vi "Coerce Value.vi"(8 "error in (no error)":errorcluster, 9 "Value":variant, 10 "ParamTags":T1, 11 "Rigol DG822 Square in":refnum<class "Rigol DG822 Square.lvclass">) -> (0 "error out":errorcluster, 1 "Coerced Value":variant, 3 "Rigol DG822 Square out":refnum<class "Rigol DG822 Square.lvclass">)   [LabVIEW 2021, in "Rigol DG822 UI.lvlib" / "Rigol DG822 Square.lvlib" / "Rigol DG822 Square.lvclass"]
uses:
  Rigol DG822 Square.lvclass
  Rigol DG822 UI/lib/controls.llb/WaveformParamTags.ctl
  Rigol DG822 UI/lib/controls.llb/FreqUnit.ctl
  Rigol DG822 UI/lib/controls.llb/PeriodUnit.ctl
  Rigol DG822 Square.lvclass/Rigol DG822 Square.ctl
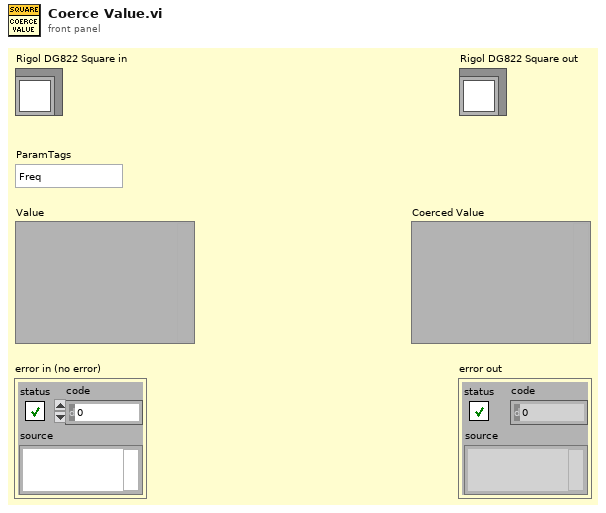
[diagram p1: front panel]
types:
  T1 = typedef "WaveformParamTags.ctl" = enum16{"Freq", "Period", "Ampl", "HighL", "Offset", "LowL", "Phase", "Duty", "Width", "RisEdge", "FallEdge"}
  T2 = typedef "FreqUnit.ctl" = enum32{"No Selection", "MHz", "kHz", "Hz", "mHz", "uHz"}
  T3 = cluster{"Freq":dbl, "FreqUnit":T2, "FreqUnitPrecision":dbl}
  T4 = typedef "PeriodUnit.ctl" = enum32{"No Selection", "s", "ms", "us", "ns"}
  T5 = cluster{"Period":dbl, "PeriodUnit":T4, "PeriodUnitPrecision":dbl}
  T6 = cluster{"Ampl":dbl, "AmplUnit":enum32{"No Selection", "Vpp", "mVpp"}, "AmplUnitPrecision":dbl}
  T7 = cluster{"HighL":dbl, "HighLUnit":enum32{"No Selection", "V", "mV"}, "HighLUnitPrecision":dbl}
  T8 = cluster{"Offset":dbl, "OffsetUnit":enum32{"No Selection", "Vdc", "mVdc"}, "OffsetUnitPrecision":dbl}
  T9 = cluster{"LowL":dbl, "LowLUnit":enum32{"No Selection", "V", "mV"}, "LowLUnitPrecision":dbl}
  T10 = cluster{"Phase":dbl, "PhaseUnit":enum32{"°"}, "PhaseUnitPrecision":dbl}
  T11 = cluster{"Duty":dbl, "DutyUnit":enum32{"%"}, "DutyUnitPrcs":dbl}
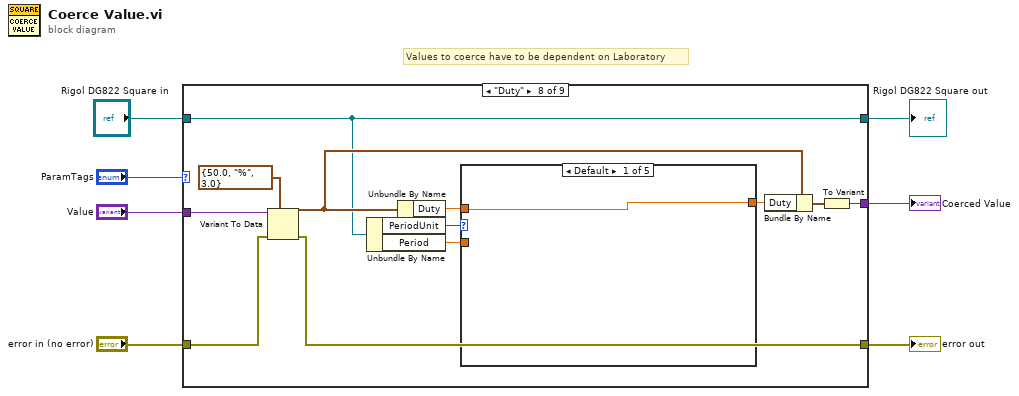
[diagram p0: block diagram]
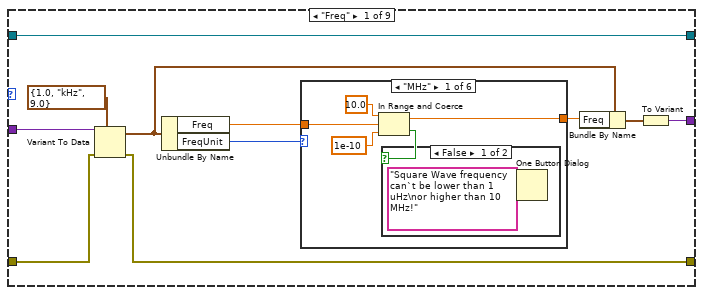
[diagram p2: hidden frame]
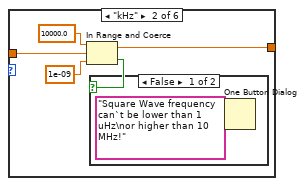
[diagram p4: hidden frame]
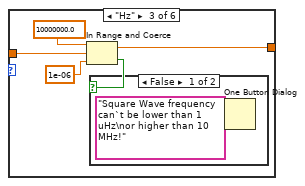
[diagram p6: hidden frame]
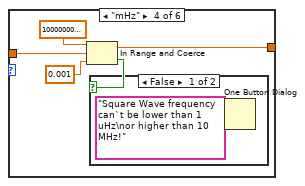
[diagram p8: hidden frame]
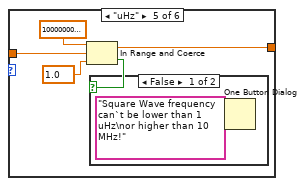
[diagram p10: hidden frame]
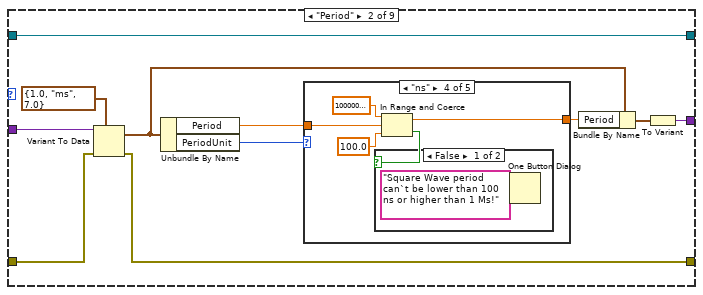
[diagram p13: hidden frame]
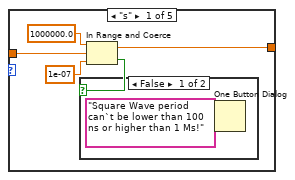
[diagram p14: hidden frame]
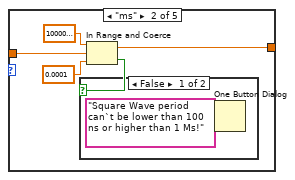
[diagram p16: hidden frame]
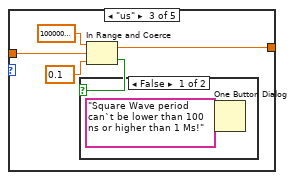
[diagram p18: hidden frame]
diagram:
  # "Values to coerce have to be dependent on Laboratory"
  n1 = case shown="\"Duty\"" "ParamTags" {
    tunnel: "Value" -> [w14 w57 w93 w119 w167 w233 w279 w296 w362]
    tunnel: "error in (no error)" -> [w12 w53 w90 w117 w165 w231 w276 w294 w361]
    tunnel: [w11 w52 w89 w116 w164 w230 w275 w293 w361] -> w4
    tunnel: [w9 w50 w87 w114 w162 w228 w273 w291 w362] -> w1
    tunnel: "Rigol DG822 Square in" -> [w8 w54 w91 w112 w160 w227 w277 w289 w363]
    tunnel: [w8 w54 w91 w112 w160 w227 w277 w289 w363] -> w2
    frame "Freq" {
      n2 = Variant To Data(error in=w12, type=T3 {"Freq"=1.0, "FreqUnit"=enum."kHz", "FreqUnitPrecision"=9.0} ("Freq"), Variant=w14) -> (data=w13:T3, error out=w11:errorcluster)
      n3 = Unbundle By Name(w13) -> ("Freq"=w17:dbl, "FreqUnit"=w18:T2)
      n4 = case shown="\"MHz\"" w18 {
        tunnel: [w20 w26 w32 w38 w44 w49] -> w16
        tunnel: w17 -> [w21 w27 w33 w39 w45 w49]
        frame "MHz" {
          n5 = In Range and Coerce(upper limit=10.0, x=w21, lower limit=1e-10 ("t")) -> (coerced(x)=w20:dbl, In Range?=w19:bool)
          n6 = case shown="False" w19 {
            frame False {
              n7 = One Button Dialog(message="Square Wave frequency can`t be lower than 1 uHz\nor higher than 10 MHz!") -> ()  [unwired: 1 in, 1 out]
            }
            frame True {
            }
          }
        }
        frame "kHz" {
          n8 = In Range and Coerce(upper limit=10000.0, x=w27, lower limit=1e-09 ("t")) -> (coerced(x)=w26:dbl, In Range?=w25:bool)
          n9 = case shown="False" w25 {
            frame False {
              n10 = One Button Dialog(message="Square Wave frequency can`t be lower than 1 uHz\nor higher than 10 MHz!") -> ()  [unwired: 1 in, 1 out]
            }
            frame True {
            }
          }
        }
        frame "Hz" {
          n11 = In Range and Coerce(upper limit=10000000.0, x=w33, lower limit=1e-06 ("t")) -> (coerced(x)=w32:dbl, In Range?=w31:bool)
          n12 = case shown="False" w31 {
            frame False {
              n13 = One Button Dialog(message="Square Wave frequency can`t be lower than 1 uHz\nor higher than 10 MHz!") -> ()  [unwired: 1 in, 1 out]
            }
            frame True {
            }
          }
        }
        frame "mHz" {
          n14 = In Range and Coerce(upper limit=10000000000.0, x=w39, lower limit=0.001 ("t")) -> (coerced(x)=w38:dbl, In Range?=w37:bool)
          n15 = case shown="False" w37 {
            frame False {
              n16 = One Button Dialog(message="Square Wave frequency can`t be lower than 1 uHz\nor higher than 10 MHz!") -> ()  [unwired: 1 in, 1 out]
            }
            frame True {
            }
          }
        }
        frame "uHz" {
          n17 = In Range and Coerce(upper limit=10000000000000.0, x=w45, lower limit=1.0 ("t")) -> (coerced(x)=w44:dbl, In Range?=w43:bool)
          n18 = case shown="False" w43 {
            frame False {
              n19 = One Button Dialog(message="Square Wave frequency can`t be lower than 1 uHz\nor higher than 10 MHz!") -> ()  [unwired: 1 in, 1 out]
            }
            frame True {
            }
          }
        }
        frame Default {
        }
      }
      n20 = Bundle By Name(cluster=w13, "Freq"=w16) -> (w10:T3)
      n21 = To Variant(anything=w10) -> (Variant=w9:variant)
    }
    frame "Period" {
      n22 = Variant To Data(error in=w53, type=T5 {"Period"=1.0, "PeriodUnit"=enum."ms", "PeriodUnitPrecision"=7.0} ("Period"), Variant=w57) -> (data=w56:T5, error out=w52:errorcluster)
      n23 = Unbundle By Name(w56) -> ("Period"=w59:dbl, "PeriodUnit"=w60:T4)
      n24 = case shown="\"ns\"" w60 {
        tunnel: [w62 w68 w74 w80 w85] -> w58
        tunnel: w59 -> [w63 w69 w75 w81 w85]
        frame "s" {
          n25 = In Range and Coerce(upper limit=1000000.0, x=w63, lower limit=1e-07 ("t")) -> (coerced(x)=w62:dbl, In Range?=w61:bool)
          n26 = case shown="False" w61 {
            frame False {
              n27 = One Button Dialog(message="Square Wave period can`t be lower than 100 ns or higher than 1 Ms!") -> ()  [unwired: 1 in, 1 out]
            }
            frame True {
            }
          }
        }
        frame "ms" {
          n28 = In Range and Coerce(upper limit=1000000000.0, x=w69, lower limit=0.0001 ("t")) -> (coerced(x)=w68:dbl, In Range?=w67:bool)
          n29 = case shown="False" w67 {
            frame False {
              n30 = One Button Dialog(message="Square Wave period can`t be lower than 100 ns or higher than 1 Ms!") -> ()  [unwired: 1 in, 1 out]
            }
            frame True {
            }
          }
        }
        frame "us" {
          n31 = In Range and Coerce(upper limit=1000000000000.0, x=w75, lower limit=0.1 ("t")) -> (coerced(x)=w74:dbl, In Range?=w73:bool)
          n32 = case shown="False" w73 {
            frame False {
              n33 = One Button Dialog(message="Square Wave period can`t be lower than 100 ns or higher than 1 Ms!") -> ()  [unwired: 1 in, 1 out]
            }
            frame True {
            }
          }
        }
        frame "ns" {
          n34 = In Range and Coerce(upper limit=1000000000000000.0, x=w81, lower limit=100.0 ("t")) -> (coerced(x)=w80:dbl, In Range?=w79:bool)
          n35 = case shown="False" w79 {
            frame False {
              n36 = One Button Dialog(message="Square Wave period can`t be lower than 100 ns or higher than 1 Ms!") -> ()  [unwired: 1 in, 1 out]
            }
            frame True {
            }
          }
        }
        frame Default {
        }
      }
      n37 = Bundle By Name(cluster=w56, "Period"=w58) -> (w51:T5)
      n38 = To Variant(anything=w51) -> (Variant=w50:variant)
    }
    frame "Ampl" {
      n39 = Variant To Data(error in=w90, type=T6 {"Ampl"=5.0, "AmplUnit"=enum."Vpp", "AmplUnitPrecision"=4.0} ("Ampl"), Variant=w93) -> (data=w92:T6, error out=w89:errorcluster)
      n40 = Unbundle By Name(w92) -> ("Ampl"=w95:dbl, "AmplUnit"=w96:enum32{"No Selection", "Vpp", "mVpp"})
      n41 = case shown="\"Vpp\"" w96 {
        tunnel: [w99 w105 w109] -> w94
        tunnel: w95 -> [w100 w106 w109]
        frame "Vpp" {
          n42 = In Range and Coerce(upper limit=10.0, x=w100, lower limit=0.002 ("t")) -> (coerced(x)=w99:dbl, In Range?=w97:bool)
          n43 = case shown="False" w97 {
            frame False {
              n44 = One Button Dialog(message="Amplitude can`t be lower than 2 mVpp\nor higher than 10 Vpp!") -> ()  [unwired: 1 in, 1 out]
            }
            frame True {
            }
          }
        }
        frame "mVpp" {
          n45 = In Range and Coerce(upper limit=10000.0, x=w106, lower limit=2.0 ("t")) -> (coerced(x)=w105:dbl, In Range?=w103:bool)
          n46 = case shown="False" w103 {
            frame False {
              n47 = One Button Dialog(message="Amplitude can`t be lower than 2 mVpp\nor higher than 10 Vpp!") -> ()  [unwired: 1 in, 1 out]
            }
            frame True {
            }
          }
        }
        frame Default {
        }
      }
      n48 = Bundle By Name(cluster=w92, "Ampl"=w94) -> (w88:T6)
      n49 = To Variant(anything=w88) -> (Variant=w87:variant)
    }
    frame "HighL" {
      n50 = Variant To Data(error in=w117, type=T7 {"HighL"=2.5, "HighLUnit"=enum."V", "HighLUnitPrecision"=4.0} ("HighL"), Variant=w119) -> (data=w118:T7, error out=w116:errorcluster)
      n51 = Unbundle By Name(w118) -> ("HighL"=w121:dbl, "HighLUnit"=w122:enum32{"No Selection", "V", "mV"})
      n52 = Unbundle By Name(w112) -> ("LowL"=w111:dbl, "LowLUnit"=w110:enum32{"No Selection", "V", "mV"})
      n53 = case shown="\"V\"" w122 {
        tunnel: [w127 w144 w157] -> w120
        tunnel: w121 -> [w128 w145 w157]
        tunnel: w111 -> [w123 w140 _]
        tunnel: w110 -> [w125 w142 _]
        frame "V" {
          n54 = case shown="\"V\"" w125 {
            tunnel: [w130 w136 w138] -> w124
            tunnel: w123 -> [w132 w137 w138]
            frame "V" {
              n55 = Add(x=w132, y=0.002 ("upper limit")) -> (x+y=w130:dbl)
            }
            frame "mV" {
              n56 = Divide(x=w137, y=1000.0) -> (x/y=w135:dbl)
              n57 = Add(x=w135, y=0.002 ("upper limit")) -> (x+y=w136:dbl)
            }
            frame Default {
            }
          }
          n58 = In Range and Coerce(upper limit=5.0, x=w128, lower limit=w124) -> (coerced(x)=w127:dbl, In Range?=w126:bool)
          n59 = case shown="False" w126 {
            frame False {
              n60 = One Button Dialog(message="HighL can`t be higher than 5 V or less than 2 mV higher than LowL!\n") -> ()  [unwired: 1 in, 1 out]
            }
            frame True {
            }
          }
        }
        frame "mV" {
          n61 = case shown="\"mV\"" w142 {
            tunnel: [w150 w154 w155] -> w141
            tunnel: w140 -> [w149 w152 w155]
            frame "V" {
              n62 = Multiply(x=w149, y=1000.0) -> (x*y=w147:dbl)
              n63 = Add(x=w147, y=2.0 ("upper limit")) -> (x+y=w150:dbl)
            }
            frame "mV" {
              n64 = Add(x=w152, y=2.0 ("upper limit")) -> (x+y=w154:dbl)
            }
            frame Default {
            }
          }
          n65 = In Range and Coerce(upper limit=5000.0, x=w145, lower limit=w141) -> (coerced(x)=w144:dbl, In Range?=w143:bool)
          n66 = case shown="False" w143 {
            frame False {
              n67 = One Button Dialog(message="HighL can`t be higher than 5 V or less than 2 mV higher than LowL!\n") -> ()  [unwired: 1 in, 1 out]
            }
            frame True {
            }
          }
        }
        frame Default {
        }
      }
      n68 = Bundle By Name(cluster=w118, "HighL"=w120) -> (w115:T7)
      n69 = To Variant(anything=w115) -> (Variant=w114:variant)
    }
    frame "Offset" {
      n70 = Variant To Data(error in=w165, type=T8 {"Offset"=0.0, "OffsetUnit"=enum."Vdc", "OffsetUnitPrecision"=4.0} ("Offset"), Variant=w167) -> (data=w166:T8, error out=w164:errorcluster)
      n71 = Unbundle By Name(w166) -> ("Offset"=w169:dbl, "OffsetUnit"=w170:enum32{"No Selection", "Vdc", "mVdc"})
      n72 = Unbundle By Name(w160) -> ("Ampl"=w159:dbl, "AmplUnit"=w158:enum32{"No Selection", "Vpp", "mVpp"})
      n73 = case shown="\"mVdc\"" w170 {
        tunnel: [w176 w202 w223] -> w168
        tunnel: w169 -> [w177 w203 w223]
        tunnel: w159 -> [w173 w199 _]
        tunnel: w158 -> [w174 w200 _]
        frame "Vdc" {
          n74 = case shown="\"Vpp\"" w174 {
            tunnel: w173 -> [w184 w192 _]
            tunnel: [w179 w187 5.0] -> w172
            tunnel: [w178 w186 -5.0] -> w171
            frame "Vpp" {
              w180 = 2.0 ("t")
              n75 = Add(x=w184, y=-10.0 ("t")) -> (x+y=w182:dbl)
              n76 = Subtract(x=10.0 ("t"), y=w184) -> (x-y=w181:dbl)
              n77 = Divide(x=w182, y=w180) -> (x/y=w178:dbl)
              n78 = Divide(x=w181, y=w180) -> (x/y=w179:dbl)
            }
            frame "mVpp" {
              w188 = 2000.0 ("t")
              n79 = Add(x=w192, y=-10000.0 ("t")) -> (x+y=w190:dbl)
              n80 = Subtract(x=10000.0 ("t"), y=w192) -> (x-y=w189:dbl)
              n81 = Divide(x=w190, y=w188) -> (x/y=w186:dbl)
              n82 = Divide(x=w189, y=w188) -> (x/y=w187:dbl)
            }
            frame Default {
            }
          }
          n83 = In Range and Coerce(upper limit=w172, x=w177, lower limit=w171) -> (coerced(x)=w176:dbl, In Range?=w175:bool)
          n84 = case shown="False" w175 {
            frame False {
              n85 = One Button Dialog(message="Offset upper and lower limit can`t exceed (10 - Ampl)/2 value") -> ()  [unwired: 1 in, 1 out]
            }
            frame True {
            }
          }
        }
        frame "mVdc" {
          n86 = case shown="\"Vpp\"" w200 {
            tunnel: w199 -> [w210 w218 _]
            tunnel: [w205 w213 5.0] -> w198
            tunnel: [w204 w212 -5.0] -> w197
            frame "Vpp" {
              w206 = 0.002 ("t")
              n87 = Add(x=w210, y=-10.0 ("t")) -> (x+y=w208:dbl)
              n88 = Subtract(x=10.0 ("t"), y=w210) -> (x-y=w207:dbl)
              n89 = Divide(x=w208, y=w206) -> (x/y=w204:dbl)
              n90 = Divide(x=w207, y=w206) -> (x/y=w205:dbl)
            }
            frame "mVpp" {
              w214 = 2.0 ("t")
              n91 = Add(x=w218, y=-10000.0 ("t")) -> (x+y=w216:dbl)
              n92 = Subtract(x=10000.0 ("t"), y=w218) -> (x-y=w215:dbl)
              n93 = Divide(x=w216, y=w214) -> (x/y=w212:dbl)
              n94 = Divide(x=w215, y=w214) -> (x/y=w213:dbl)
            }
            frame Default {
            }
          }
          n95 = In Range and Coerce(upper limit=w198, x=w203, lower limit=w197) -> (coerced(x)=w202:dbl, In Range?=w201:bool)
          n96 = case shown="False" w201 {
            frame False {
              n97 = One Button Dialog(message="Offset upper and lower limit can`t exceed (10 - Ampl)/2 value") -> ()  [unwired: 1 in, 1 out]
            }
            frame True {
            }
          }
        }
        frame Default {
        }
      }
      n98 = Bundle By Name(cluster=w166, "Offset"=w168) -> (w163:T8)
      n99 = To Variant(anything=w163) -> (Variant=w162:variant)
    }
    frame "LowL" {
      n100 = Variant To Data(error in=w231, type=T9 {"LowL"=-2.5, "LowLUnit"=enum."V", "LowLUnitPrecision"=4.0} ("LowL"), Variant=w233) -> (data=w232:T9, error out=w230:errorcluster)
      n101 = Unbundle By Name(w232) -> ("LowL"=w235:dbl, "LowLUnit"=w236:enum32{"No Selection", "V", "mV"})
      n102 = Unbundle By Name(w227) -> ("HighL"=w226:dbl, "HighLUnit"=w225:enum32{"No Selection", "V", "mV"})
      n103 = case shown="\"mV\"" w236 {
        tunnel: [w242 w259 w271] -> w234
        tunnel: w235 -> [w243 w260 w271]
        tunnel: w226 -> [w239 w256 _]
        tunnel: w225 -> [w240 w257 _]
        frame "V" {
          n104 = case shown="\"mV\"" w240 {
            tunnel: [w244 w250 w252] -> w237
            tunnel: w239 -> [w246 w251 w252]
            frame "V" {
              n105 = Subtract(x=w246, y=0.002 ("upper limit")) -> (x-y=w244:dbl)
            }
            frame "mV" {
              n106 = Divide(x=w251, y=1000.0) -> (x/y=w249:dbl)
              n107 = Subtract(x=w249, y=0.002 ("upper limit")) -> (x-y=w250:dbl)
            }
            frame Default {
            }
          }
          n108 = In Range and Coerce(upper limit=w237, x=w243, lower limit=-5.0 ("upper limit")) -> (coerced(x)=w242:dbl, In Range?=w241:bool)
          n109 = case shown="False" w241 {
            frame False {
              n110 = One Button Dialog(message="LowL can`t be lower  than -5 V or less than 2 mV lower than HighL!") -> ()  [unwired: 1 in, 1 out]
            }
            frame True {
            }
          }
        }
        frame "mV" {
          n111 = case shown="\"V\"" w257 {
            tunnel: [w264 w268 w269] -> w254
            tunnel: w256 -> [w263 w266 w269]
            frame "V" {
              n112 = Multiply(x=w263, y=1000.0) -> (x*y=w261:dbl)
              n113 = Subtract(x=w261, y=2.0 ("upper limit")) -> (x-y=w264:dbl)
            }
            frame "mV" {
              n114 = Subtract(x=w266, y=2.0 ("upper limit")) -> (x-y=w268:dbl)
            }
            frame Default {
            }
          }
          n115 = In Range and Coerce(upper limit=w254, x=w260, lower limit=-5000.0 ("upper limit")) -> (coerced(x)=w259:dbl, In Range?=w258:bool)
          n116 = case shown="False" w258 {
            frame False {
              n117 = One Button Dialog(message="LowL can`t be lower  than -5 V or less than 2 mV lower than HighL!") -> ()  [unwired: 1 in, 1 out]
            }
            frame True {
            }
          }
        }
        frame Default {
        }
      }
      n118 = Bundle By Name(cluster=w232, "LowL"=w234) -> (w229:T9)
      n119 = To Variant(anything=w229) -> (Variant=w228:variant)
    }
    frame "Phase" {
      n120 = Variant To Data(error in=w276, type=T10 {"Phase"=0.0, "PhaseUnit"=enum."°", "PhaseUnitPrecision"=3.0} ("Phase"), Variant=w279) -> (data=w278:T10, error out=w275:errorcluster)
      n121 = Unbundle By Name(w278) -> ("Phase"=w281:dbl, "PhaseUnit"=w282:enum32{"°"})
      n122 = case shown="\"°\"" w282 {
        tunnel: [w283 w284] -> w280
        tunnel: w281 -> [w283 w285]
        frame Default {
        }
        frame "°" {
          n123 = Quotient & Remainder(x=w285, y=360.0) -> (x-y*floor(x/y)=w284:dbl)  [unwired: 1 out]
        }
      }
      n124 = Bundle By Name(cluster=w278, "Phase"=w280) -> (w274:T10)
      n125 = To Variant(anything=w274) -> (Variant=w273:variant)
    }
    frame "Duty" {
      n126 = Variant To Data(error in=w294, type=T11 {"Duty"=50.0, "DutyUnit"=enum."%", "DutyUnitPrcs"=3.0} ("Duty"), Variant=w296) -> (data=w295:T11, error out=w293:errorcluster)
      n127 = Unbundle By Name(w289) -> ("PeriodUnit"=w288:enum32{"No Selection", "s", "ms", "us", "ns"}, "Period"=w287:dbl)
      n128 = Unbundle By Name(w295) -> ("Duty"=w298:dbl)
      n129 = case shown="Default" w288 {
        tunnel: [w299 w308 w325 w342 w354] -> w297
        tunnel: w298 -> [w299 w307 w324 w341 w353]
        tunnel: w287 -> [_ w302 w319 w336 _]
        frame Default {
        }
        frame "ns" {
          w301 = 2000.0 ("lower limit")
          n130 = Multiply(x=100.0 ("y"), y=w302) -> (x*y=w309:dbl)
          n131 = Multiply(x=w307, y=w302) -> (x*y=w311:dbl)
          n132 = Divide(x=w301, y=w302) -> (x/y=w303:dbl)
          n133 = Subtract(x=w309, y=w301) -> (x-y=w300:dbl)
          n134 = Divide(x=w300, y=w302) -> (x/y=w304:dbl)
          n135 = In Range and Coerce(upper limit=w300, x=w311, lower limit=w301) -> (coerced(x)=w310:dbl, In Range?=w305:bool)
          n136 = case shown="False" w305 {
            tunnel: w303 -> [w315 _]
            tunnel: w304 -> [w312 _]
            frame False {
              w313 = "%" ("input 2")
              n137 = Format Into String(format string="Duty Cycle can`t be lower than %.3f %s\nor higher than %.3f %s!" ("message"), w315, w313, w312, w313) -> (resulting string=w316:string)  [unwired: 2 in, 1 out]
              n138 = One Button Dialog(message=w316) -> ()  [unwired: 1 in, 1 out]
            }
            frame True {
            }
          }
          n139 = Divide(x=w310, y=w302) -> (x/y=w308:dbl)
        }
        frame "us" {
          w318 = 2.0 ("lower limit")
          n140 = Multiply(x=100.0 ("y"), y=w319) -> (x*y=w326:dbl)
          n141 = Multiply(x=w324, y=w319) -> (x*y=w328:dbl)
          n142 = Divide(x=w318, y=w319) -> (x/y=w320:dbl)
          n143 = Subtract(x=w326, y=w318) -> (x-y=w317:dbl)
          n144 = Divide(x=w317, y=w319) -> (x/y=w321:dbl)
          n145 = In Range and Coerce(upper limit=w317, x=w328, lower limit=w318) -> (coerced(x)=w327:dbl, In Range?=w322:bool)
          n146 = case shown="False" w322 {
            tunnel: w320 -> [w332 _]
            tunnel: w321 -> [w329 _]
            frame False {
              w330 = "%" ("input 2")
              n147 = Format Into String(format string="Duty Cycle can`t be lower than %.3f %s\nor higher than %.3f %s!" ("message"), w332, w330, w329, w330) -> (resulting string=w333:string)  [unwired: 2 in, 1 out]
              n148 = One Button Dialog(message=w333) -> ()  [unwired: 1 in, 1 out]
            }
            frame True {
            }
          }
          n149 = Divide(x=w327, y=w319) -> (x/y=w325:dbl)
        }
        frame "ms" {
          w335 = 0.002 ("lower limit")
          n150 = Multiply(x=100.0 ("y"), y=w336) -> (x*y=w343:dbl)
          n151 = Multiply(x=w341, y=w336) -> (x*y=w345:dbl)
          n152 = Divide(x=w335, y=w336) -> (x/y=w337:dbl)
          n153 = Subtract(x=w343, y=w335) -> (x-y=w334:dbl)
          n154 = Divide(x=w334, y=w336) -> (x/y=w338:dbl)
          n155 = In Range and Coerce(upper limit=w334, x=w345, lower limit=w335) -> (coerced(x)=w344:dbl, In Range?=w339:bool)
          n156 = case shown="False" w339 {
            tunnel: w337 -> [w349 _]
            tunnel: w338 -> [w346 _]
            frame False {
              w347 = "%" ("input 2")
              n157 = Format Into String(format string="Duty Cycle can`t be lower than %.3f %s\nor higher than %.3f %s!" ("message"), w349, w347, w346, w347) -> (resulting string=w350:string)  [unwired: 2 in, 1 out]
              n158 = One Button Dialog(message=w350) -> ()  [unwired: 1 in, 1 out]
            }
            frame True {
            }
          }
          n159 = Divide(x=w344, y=w336) -> (x/y=w342:dbl)
        }
        frame "s" {
          w352 = 0.005 ("lower limit")
          w351 = 99.995 ("upper limit")
          n160 = In Range and Coerce(upper limit=w351, x=w353, lower limit=w352) -> (coerced(x)=w354:dbl, In Range?=w355:bool)
          n161 = case shown="False" w355 {
            tunnel: w352 -> [w359 _]
            tunnel: w351 -> [w356 _]
            frame False {
              w357 = "%" ("input 2")
              n162 = Format Into String(format string="Duty Cycle can`t be lower than %.3f %s\nor higher than %.3f %s!" ("message"), w359, w357, w356, w357) -> (resulting string=w360:string)  [unwired: 2 in, 1 out]
              n163 = One Button Dialog(message=w360) -> ()  [unwired: 1 in, 1 out]
            }
            frame True {
            }
          }
        }
      }
      n164 = Bundle By Name(cluster=w295, "Duty"=w297) -> (w292:T11)
      n165 = To Variant(anything=w292) -> (Variant=w291:variant)
    }
    frame Default {
    }
  }
  "error out" <- w4
  "Rigol DG822 Square out" <- w2
  "Coerced Value" <- w1
